vi "Get_All_Result.vi"(9 "Test_Result":bool[](array[boolean]), 10 "SN_Result":bool[](array[boolean])) -> (2 "All_Result":bool[](array[boolean]))   [LabVIEW 2018]
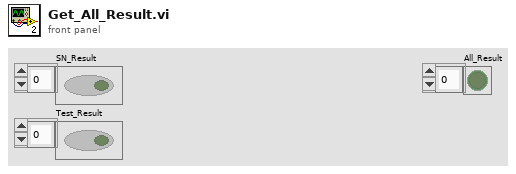
[diagram p1: front panel]
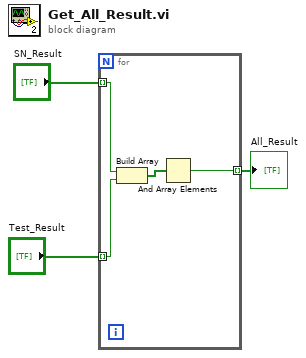
[diagram p0: block diagram]
diagram:
  n1 = for {
    tunnel: "SN_Result" -> [w7] mode=indexing
    tunnel: "Test_Result" -> [w6] mode=indexing
    tunnel: [w4] -> w1 mode=indexing
    n2 = Build Array(w7, w6) -> (w5:bool[])
    n3 = And Array Elements(Boolean array=w5) -> (logical AND=w4:bool)
  }
  "All_Result" <- w1
